vi "epics put uniformity.vi"(7 "Value In":variant, 8 "error in":errorcluster, 11 "CA in":T1) -> (0 "error out":errorcluster, 2 "Status":bool)   [LabVIEW 2022 SP3]
uses:
  Program Files/National Instruments/LabVIEW 2023/user.lib/calab/CaLab.lvlib
  Program Files/National Instruments/LabVIEW 2023/user.lib/calab/private/Put_DBL_PV.vi
  Program Files/National Instruments/LabVIEW 2023/user.lib/calab/private/Put_Boolean_PV.vi
  Program Files/National Instruments/LabVIEW 2023/user.lib/calab/private/Put_String_PV.vi
  pectus/control/ca cluster.ctl
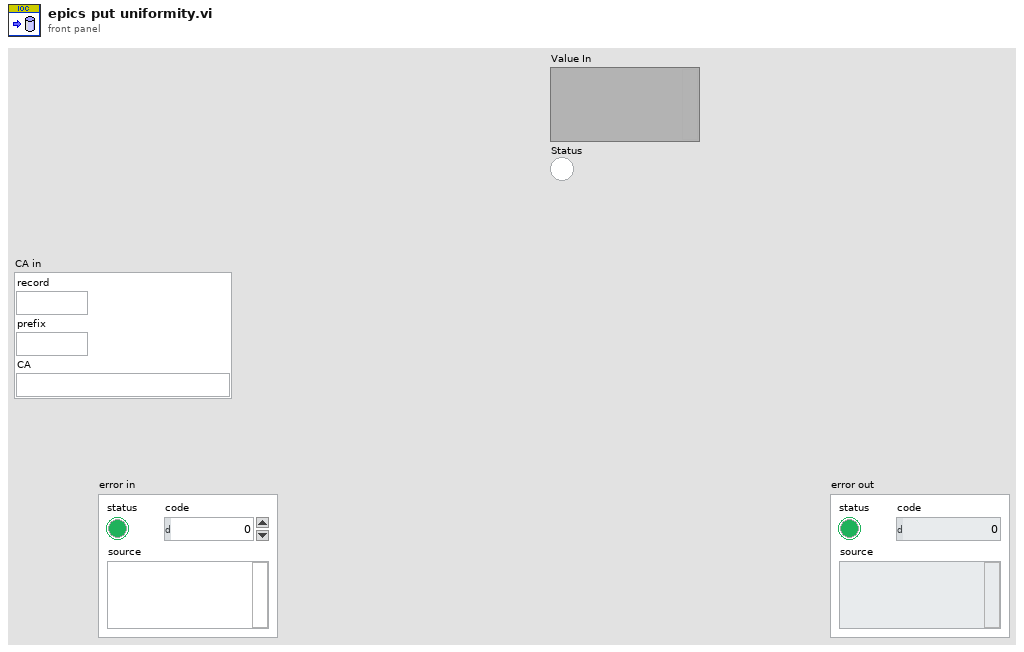
[diagram p1: front panel]
types:
  T1 = typedef "ca cluster.ctl" = cluster{"record":string, "prefix":string, "CA":string}
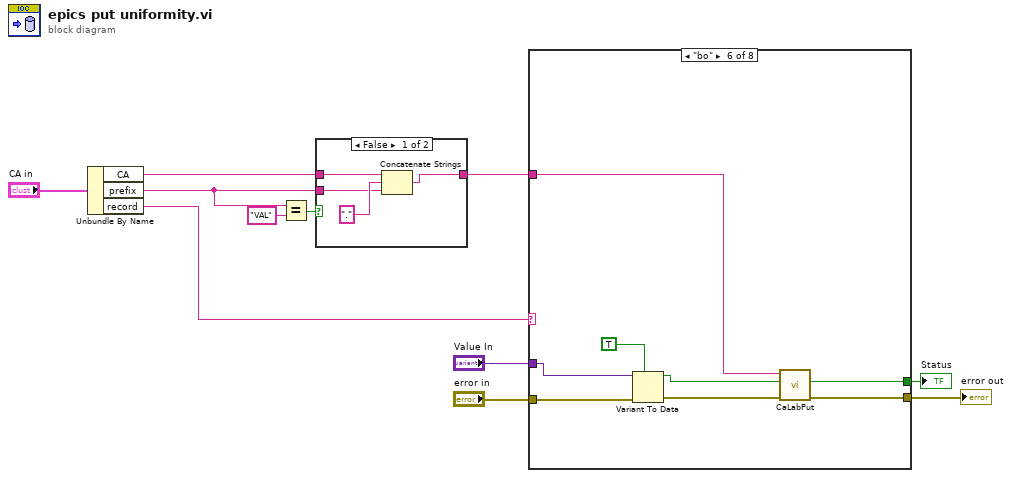
[diagram p0: block diagram]
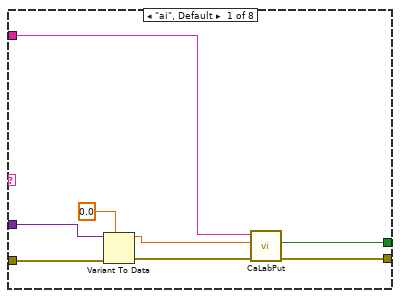
[diagram p3: hidden frame]
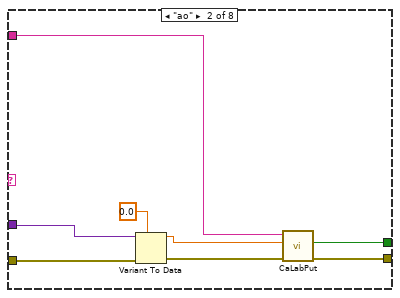
[diagram p4: hidden frame]
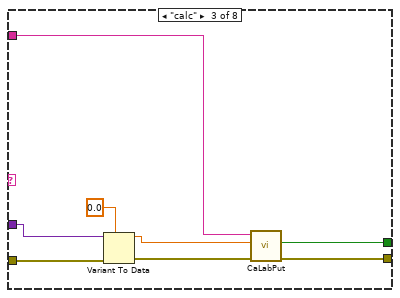
[diagram p5: hidden frame]
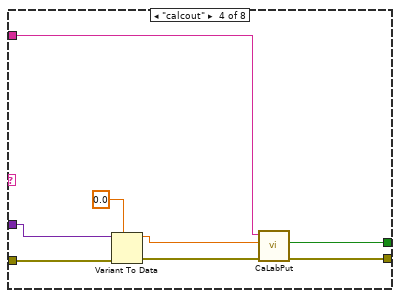
[diagram p6: hidden frame]
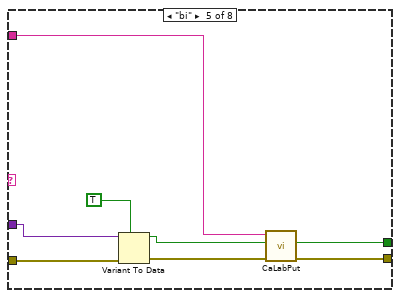
[diagram p7: hidden frame]
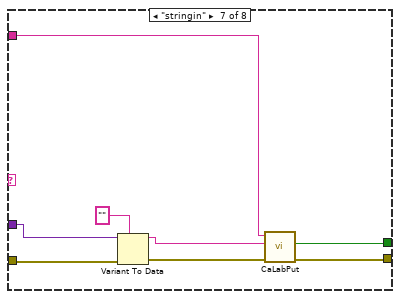
[diagram p8: hidden frame]
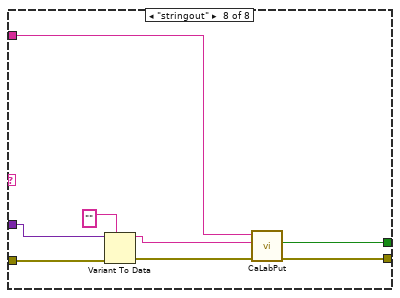
[diagram p9: hidden frame]
diagram:
  n1 = Unbundle By Name("CA in") -> ("CA"=w4:string, "prefix"=w3:string, "record"=w1:string)
  n2 = Equal?(x=w3, y="VAL") -> (x = y?=w5:bool)
  n3 = case shown="False" w5 {
    tunnel: w4 -> [w15 w16]
    tunnel: [w12 w16] -> w2
    tunnel: w3 -> [w13 _]
    frame False {
      n4 = Concatenate Strings(w15, ".", w13) -> (w12:string)
    }
    frame True {
    }
  }
  n5 = case shown="\"bo\"" w1 {
    tunnel: "Value In" -> [w22 w27 w35 w43 w52 w59 w68 w75]
    tunnel: "error in" -> [w23 w29 w38 w46 w54 w62 w69 w77]
    tunnel: [w18 w30 w37 w44 w53 w61 w67 w76] -> w9
    tunnel: w2 -> [w20 w26 w34 w42 w50 w58 w66 w74]
    tunnel: [w17 w25 w33 w41 w49 w57 w65 w73] -> w8
    frame "ai", Default {
      n6 = Variant To Data(error in=w23, type=0.0, Variant=w22) -> (data=w21:dbl, error out=w19:errorcluster)
      n7 = call-poly "CaLabPut.vi"("Error in (no error)"=w19, "Value"=w21, "PV Name"=w20) -> ("Error out"=w18:errorcluster, "Status"=w17:bool)  [unwired: 5 in, 2 out]
    }
    frame "ao" {
      n8 = Variant To Data(error in=w29, type=0.0, Variant=w27) -> (data=w32:dbl, error out=w31:errorcluster)
      n9 = call-poly "CaLabPut.vi"("Error in (no error)"=w31, "Value"=w32, "PV Name"=w26) -> ("Error out"=w30:errorcluster, "Status"=w25:bool)  [unwired: 5 in, 2 out]
    }
    frame "calc" {
      n10 = Variant To Data(error in=w38, type=0.0, Variant=w35) -> (data=w40:dbl, error out=w39:errorcluster)
      n11 = call-poly "CaLabPut.vi"("Error in (no error)"=w39, "Value"=w40, "PV Name"=w34) -> ("Error out"=w37:errorcluster, "Status"=w33:bool)  [unwired: 5 in, 2 out]
    }
    frame "calcout" {
      n12 = Variant To Data(error in=w46, type=0.0, Variant=w43) -> (data=w48:dbl, error out=w47:errorcluster)
      n13 = call-poly "CaLabPut.vi"("Error in (no error)"=w47, "Value"=w48, "PV Name"=w42) -> ("Error out"=w44:errorcluster, "Status"=w41:bool)  [unwired: 5 in, 2 out]
    }
    frame "bi" {
      n14 = Variant To Data(error in=w54, type=TRUE, Variant=w52) -> (data=w56:bool, error out=w55:errorcluster)
      n15 = call-poly "CaLabPut.vi"("Error in (no error)"=w55, "Value"=w56, "PV Name"=w50) -> ("Error out"=w53:errorcluster, "Status"=w49:bool)  [unwired: 5 in, 2 out]
    }
    frame "bo" {
      n16 = Variant To Data(error in=w62, type=TRUE, Variant=w59) -> (data=w64:bool, error out=w63:errorcluster)
      n17 = call-poly "CaLabPut.vi"("Error in (no error)"=w63, "Value"=w64, "PV Name"=w58) -> ("Error out"=w61:errorcluster, "Status"=w57:bool)  [unwired: 5 in, 2 out]
    }
    frame "stringin" {
      n18 = Variant To Data(error in=w69, type="", Variant=w68) -> (data=w71:string, error out=w70:errorcluster)
      n19 = call-poly "CaLabPut.vi"("Error in (no error)"=w70, "Value"=w71, "PV Name"=w66) -> ("Error out"=w67:errorcluster, "Status"=w65:bool)  [unwired: 5 in, 2 out]
    }
    frame "stringout" {
      n20 = Variant To Data(error in=w77, type="", Variant=w75) -> (data=w80:string, error out=w79:errorcluster)
      n21 = call-poly "CaLabPut.vi"("Error in (no error)"=w79, "Value"=w80, "PV Name"=w74) -> ("Error out"=w76:errorcluster, "Status"=w73:bool)  [unwired: 5 in, 2 out]
    }
  }
  "error out" <- w9
  "Status" <- w8
